vi "Create 2D array of text and style.vi"(0 "Find tag ?":bool, 5 "Text":string, 7 "Tags list [ ]":string[](array[string]), 9 "Tags position [ ]":i32[](array[numeric]), 11 "error in (no error)":errorcluster) -> (4 "Find tag ? duplicate":bool, 6 "Text duplicate":string, 8 "Style [ ]":T1[][](array[typedef]), 15 "error out":errorcluster)   [LabVIEW 2019]
doc: "Version 1.0\nDeveloped by Jean-Marc Simard\nCopyright © 2011, Exaprom Inc.\nAll rights reserved.\nLicense: BSD\n\nWith iTextSharp 4.1.6 (http://itextsharp.sourceforge.net)\nunder Mozilla Public License Version 1.1\n(http://www.mozilla.org/MPL/MPL-1.1.html)"
uses:
  <userlib>/Exaprom PDF/Controls/Text Controls/HTML tags.ctl
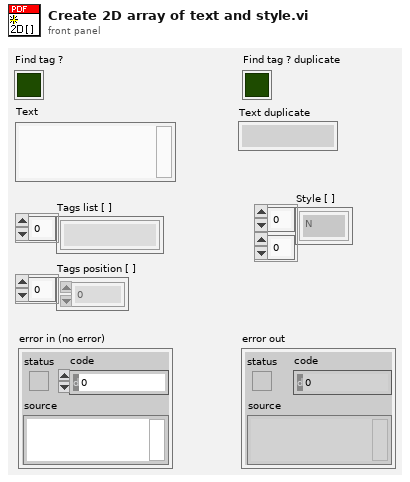
[diagram p1: front panel]
types:
  T1 = typedef "HTML tags.ctl" = enum16{"N", "b", "u", "s", "i"}
  T2 = cluster{"Text":string, "offset past match":i32, "offset past match":i32}[]
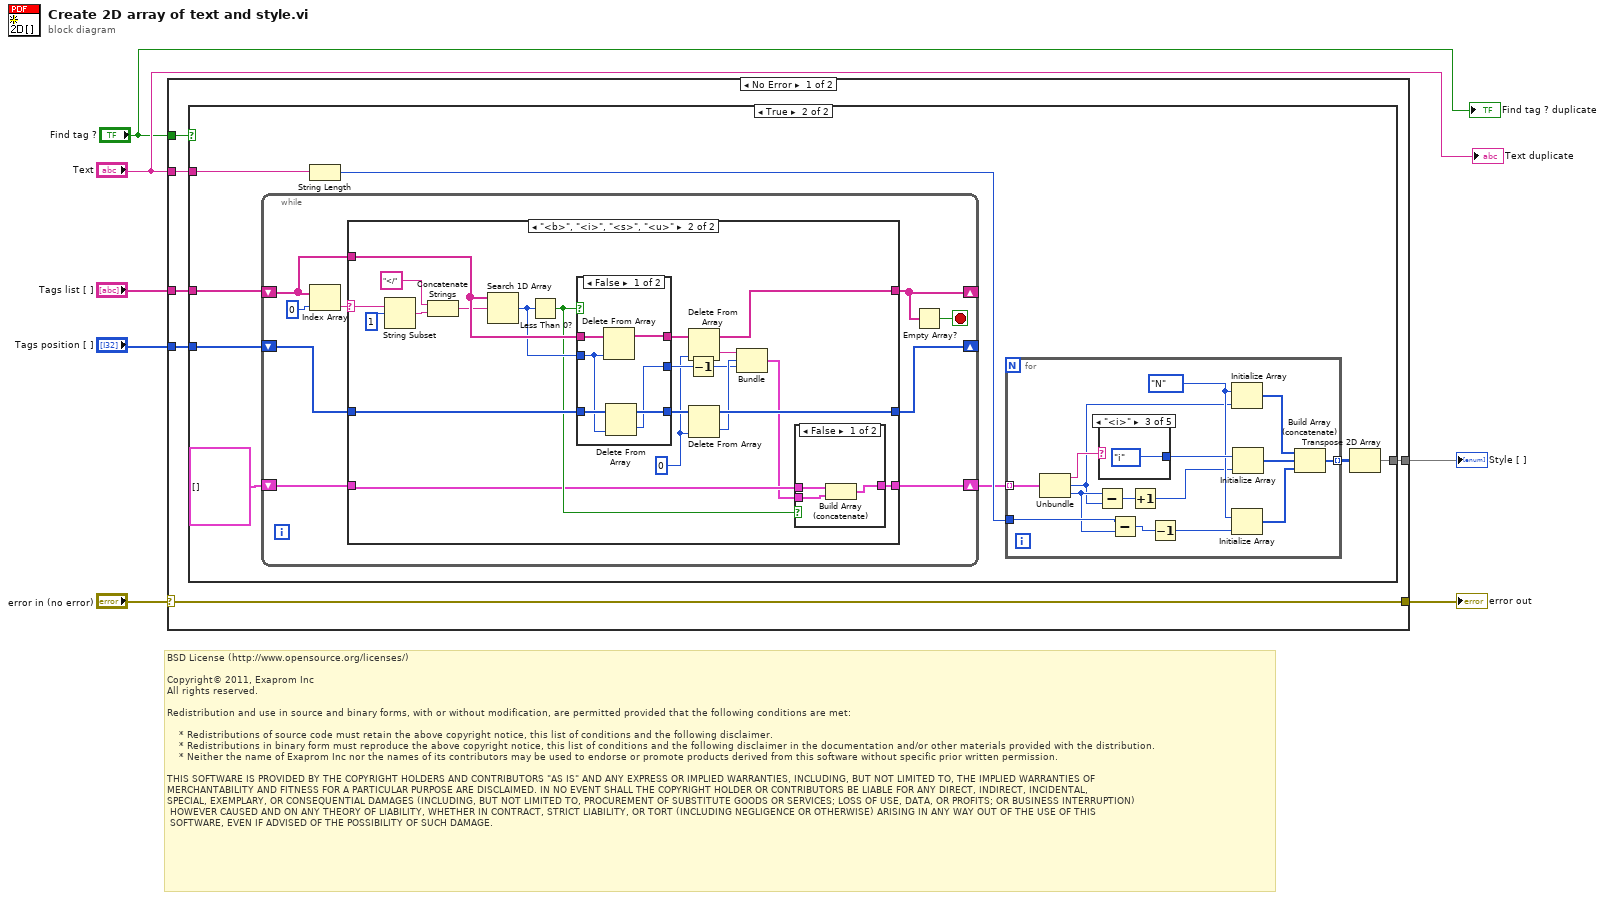
[diagram p0: block diagram]
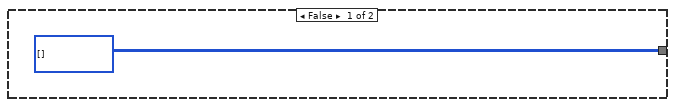
[diagram p2: hidden frame]
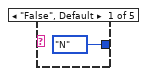
[diagram p3: hidden frame]
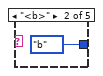
[diagram p4: hidden frame]
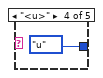
[diagram p5: hidden frame]
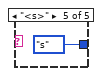
[diagram p6: hidden frame]
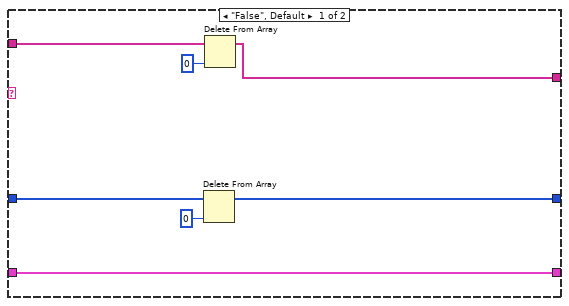
[diagram p7: hidden frame]
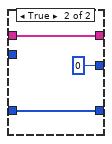
[diagram p9: hidden frame]
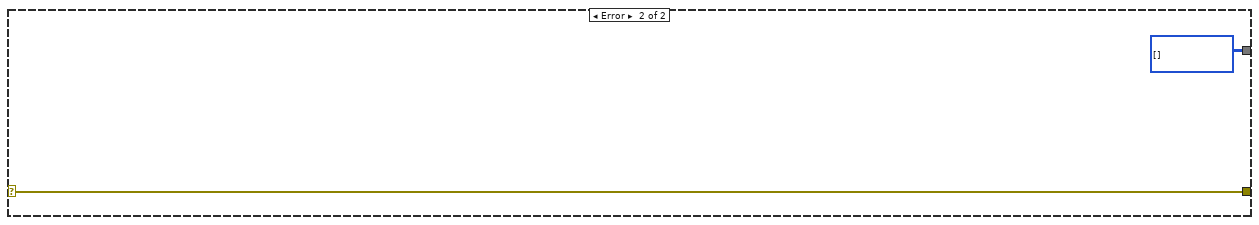
[diagram p10: hidden frame]
diagram:
  # "BSD License (http://www.opensource.org/licenses/)\n\nCopyright© 2011, Exaprom Inc\nAll rights reserved.\n\nRedistribution and use in source and binary forms, with or without modification, are permitted provided that the following conditions are met:\n\n    * Redistributions of source code must retain the above copyright notice, this list of conditions and the following disclaimer.\n    * Redistributions in binary form must reproduce the above copyright notice, this list of conditions and the following disclaimer in the documentation and/or other materials provided with the distribution.\n    * Neither the name of Exaprom Inc nor the names of its contributors may be used to endorse or promote products derived from this software without specific prior written permission.\n\nTHIS SOFTWARE IS PROVIDED BY THE COPYRIGHT HOLDERS AND CONTRIBUTORS \"AS IS\" AND ANY EXPRESS OR IMPLIED WARRANTIES, INCLUDING, BUT NOT LIMITED TO, THE IMPLIED WARRANTIES OF \nMERCHANTABILITY AND FITNESS FOR A PARTICULAR PURPOSE ARE DISCLAIMED. IN NO EVENT SHALL THE COPYRIGHT HOLDER OR CONTRIBUTORS BE LIABLE FOR ANY DIRECT, INDIRECT, INCIDENTAL,\nSPECIAL, EXEMPLARY, OR CONSEQUENTIAL DAMAGES (INCLUDING, BUT NOT LIMITED TO, PROCUREMENT OF SUBSTITUTE GOODS OR SERVICES; LOSS OF USE, DATA, OR PROFITS; OR BUSINESS INTERRUPTION)\n HOWEVER CAUSED AND ON ANY THEORY OF LIABILITY, WHETHER IN CONTRACT, STRICT LIABILITY, OR TORT (INCLUDING NEGLIGENCE OR OTHERWISE) ARISING IN ANY WAY OUT OF THE USE OF THIS\n SOFTWARE, EVEN IF ADVISED OF THE POSSIBILITY OF SUCH DAMAGE."
  n1 = case shown="No Error" "error in (no error)" {
    selector: "error in (no error)" -> [w13 w94]
    tunnel: [w13 w94] -> w7
    tunnel: "Text" -> [w12 _]
    tunnel: "Tags list [ ]" -> [w11 _]
    tunnel: "Tags position [ ]" -> [w10 _]
    tunnel: [w9 w93] -> w2
    tunnel: "Find tag ?" -> [w8 _]
    frame No Error {
      n2 = case shown="True" w8 {
        tunnel: w12 -> [_ w18]
        tunnel: w11 -> [_ w17]
        tunnel: w10 -> [_ w16]
        tunnel: [w14 w15] -> w9
        frame False {
          w14 = T1[][] [] items=["N", "b", "u", "s", "i"]
        }
        frame True {
          n3 = while {
            shift-right: [w43] -> _
            shift-left: w17 -> [w44]
            shift-right: [w48] -> _
            shift-left: w16 -> [w49]
            shift-right: [w47] -> w20
            shift-left: T2 [] -> [w46]
            stop <- w45 stop-if-true
            n4 = Index Array(array=w44, index=0) -> (element=w51:string)
            n5 = case shown="\"<b>\", \"<i>\", \"<s>\", \"<u>\"" w51 {
              selector: w51 -> [_ w67]
              tunnel: w44 -> [w58 w79]
              tunnel: w49 -> [w55 w76]
              tunnel: [w57 w74] -> w43
              tunnel: [w56 w73] -> w48
              tunnel: w46 -> [w54 w70]
              tunnel: [w54 w68] -> w47
              frame "False", Default {
                n6 = Delete From Array(array=w55, index=0) -> (array with subset deleted=w56:i32[])  [unwired: 1 in, 1 out]
                n7 = Delete From Array(array=w58, index=0) -> (array with subset deleted=w57:string[])  [unwired: 1 in, 1 out]
              }
              frame "<b>", "<i>", "<s>", "<u>" {
                w60 = 0 ("index")
                n8 = String Subset(string=w67, offset (0)=1) -> (substring=w64:string)  [unwired: 1 out]
                n9 = Concatenate Strings("</" ("substring (\"\")"), w64) -> (w63:string)
                n10 = Search 1D Array(1D array=w79, element=w63) -> (index of element=w77:i32)  [unwired: 1 out]
                n11 = Less Than 0?(x=w77) -> (x < 0?=w71:bool)
                n12 = case shown="False" w71 {
                  tunnel: w79 -> [w89 w92]
                  tunnel: [w88 w92] -> w78
                  tunnel: w77 -> [w86 _]
                  tunnel: w76 -> [w87 w91]
                  tunnel: [w85 w91] -> w75
                  tunnel: [w84 0 ("offset past match")] -> w61
                  frame False {
                    n13 = Delete From Array(array=w89, index=w86) -> (array with subset deleted=w88:string[])  [unwired: 1 in, 1 out]
                    n14 = Delete From Array(array=w87, index=w86) -> (deleted portion=w84:i32, array with subset deleted=w85:i32[])  [unwired: 1 in]
                  }
                  frame True {
                  }
                }
                n15 = Decrement(x=w61) -> (x-1=w59:i32)
                n16 = Delete From Array(array=w78, index=w60) -> (deleted portion=w72:string, array with subset deleted=w74:string[])  [unwired: 1 in]
                n17 = Delete From Array(array=w75, index=w60) -> (deleted portion=w62:i32, array with subset deleted=w73:i32[])  [unwired: 1 in]
                n18 = Bundle("Text"=w72, w62, w59) -> (w69:cluster{"Text":string, i32, i32})  [unwired: 1 out]
                n19 = case shown="False" w71 {
                  tunnel: w70 -> [w82 w83]
                  tunnel: w69 -> [w81 _]
                  tunnel: [w80 w83] -> w68
                  frame False {
                    n20 = Build Array (concatenate)(w82, w81) -> (w80:T2)
                  }
                  frame True {
                  }
                }
              }
            }
            n21 = Empty Array?(array=w43) -> (empty?=w45:bool)
          }
          n22 = String Length(string=w18) -> (length=w21:i32)
          n23 = for {
            tunnel: w20 -> [w37] mode=indexing
            tunnel: w21 -> [w32]
            tunnel: [w26] -> w22 mode=indexing
            w33 = HTML_tags."N" ("Enum")
            n24 = Unbundle(w37) -> ("Text"=w36:string, "offset past match"=w25:i32, "offset past match"=w31:i32)
            n25 = Subtract(x=w31, y=w25) -> (x-y=w34:i32)
            n26 = case shown="\"<i>\"" w36 {
              tunnel: [HTML_tags."N" ("Enum") HTML_tags."b" ("Enum") HTML_tags."i" ("Enum") HTML_tags."u" ("Enum") HTML_tags."s" ("Enum")] -> w35
              frame "False", Default {
              }
              frame "<b>" {
              }
              frame "<i>" {
              }
              frame "<u>" {
              }
              frame "<s>" {
              }
            }
            n27 = Subtract(x=w32, y=w31) -> (x-y=w30:i32)
            n28 = Increment(x=w34) -> (x+1=w24:i32)
            n29 = Decrement(x=w30) -> (x-1=w23:i32)
            n30 = Initialize Array(w33, w25) -> (w29:T1[])
            n31 = Initialize Array(w33, w23) -> (w27:T1[])
            n32 = Initialize Array(w35, w24) -> (w28:T1[])
            n33 = Build Array (concatenate)(w29, w28, w27) -> (w26:T1[])
          }
          n34 = Transpose 2D Array(2D array=w22) -> (transposed array=w15:T1[][])
        }
      }
    }
    frame Error {
      w93 = T1[][] [] items=["N", "b", "u", "s", "i"]
    }
  }
  "error out" <- w7
  "Style [ ]" <- w2
  "Text duplicate" <- "Text"
  "Find tag ? duplicate" <- "Find tag ?"
